vi "搜索所有匹配元素(2D I32).vi"(8 "error in (no error)":errorcluster caption="错误输入（无错误）", 9 "开始索引（0）":i32, 10 "元素":i32, 11 "数组":i32[][](array[numeric])) -> (0 "error out":errorcluster caption="错误输出", 1 "匹配数量":i32, 3 "匹配元素索引":cluster{"行":i32, "列":i32}[](array[cluster]))   [LabVIEW 2012]
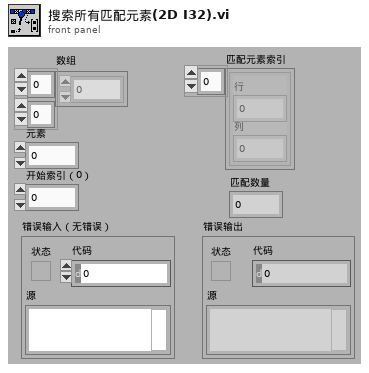
[diagram p1: front panel]
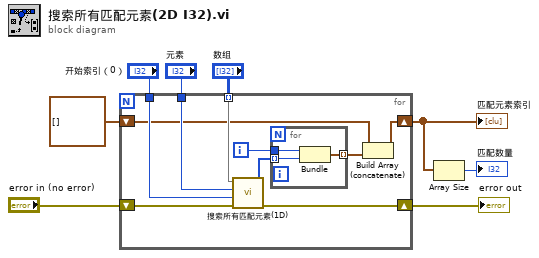
[diagram p0: block diagram]
diagram:
  n1 = for {
    tunnel: "数组" -> [w18] mode=indexing
    tunnel: "元素" -> [w17]
    tunnel: "开始索引（0）" -> [w16]
    shift-right: [w11] -> w4
    shift-left: cluster{i32, "数值":i32}[] [] -> [w13]
    shift-right: [w9] -> w1
    shift-left: "error in (no error)" -> [w10]
    i -> [w14]
    n2 = call-poly "搜索所有匹配元素(1D).vi"("error in (no error)"=w10, "开始索引（0）"=w16, "元素"=w17, "数组"=w18) -> ("error out"=w9:errorcluster, "匹配元素索引"=w15:i32[])  [unwired: 5 in, 1 out]
    n3 = for {
      tunnel: w15 -> [w21] mode=indexing
      tunnel: w14 -> [w20]
      tunnel: [w19] -> w12 mode=indexing
      n4 = Bundle(w20, "数值"=w21) -> (w19:cluster{i32, "数值":i32})  [unwired: 1 in]
    }
    n5 = Build Array (concatenate)(w13, w12) -> (w11:cluster{i32, "数值":i32}[])
  }
  "error out" <- w1
  "匹配元素索引" <- w4
  n6 = Array Size(array=w4) -> (size(s)=→"匹配数量":i32)
